vi "Module Init.vi"(8 "error in (no error)":errorcluster, 11 "ValveControlModule in":refnum<class "ValveControlModule.lvclass">) -> (0 "error out":errorcluster, 3 "ValveControlModule out":refnum<class "ValveControlModule.lvclass">)   [LabVIEW 2020, in "VolatusControl.lvlib" / "ValveControlModule.lvclass"]
uses:
  ValveControlModule.lvclass
  C:/dev/lv20CE/relink/lv-volatus/Volatus/Module/Module.lvclass
  Volatus/Remote Messaging Module/Message Registration.ctl
  lv-vecto/Vecto/Group/Group.lvclass
  C:/dev/lv20CE/relink/lv-vecto/Vecto/GroupAbstract/GroupAbstract.lvclass
  VolatusConfig/Meta Type.ctl
  Volatus/Module/Module.lvclass/Module.ctl
  VolatusConfig/VolatusConfigElement/VolatusConfigElement.lvclass/VolatusConfigElement.ctl
  ValveControlModule.lvclass/ValveControlModule.ctl
  Volatus/Module/Config.vi
  VolatusConfig/VolatusConfigElement/Element.vi
  VolatusConfig/Task/Task.lvclass
  C:/dev/lv20CE/relink/lv-volatus/VolatusConfig/VolatusConfigElement/VolatusConfigElement.lvclass
  lv-cdm/CDM-Config/Config Lookup/Match Meta.vi
  lv-cdm/CDM-Config/Config Element/Owner.vi
  lv-cdm/CDM-Config/Config Manager/Lookup Descendant.vi
  lv-cdm/CDM-Config/Config Filter/Config Lookup.lvclass
  lv-cdm/CDM-Config/Config Element/Config Element.lvclass
  Volatus/Module/Module.lvclass
  Volatus/Remote Messaging Module/Remote Messaging Module.lvclass
  VolatusConfig/Group/Group.lvclass
  VolatusData/Data Processor Module/Data Processor Module.lvclass
  C:/dev/lv20CE/relink/lv-volatus/VolatusControl/ValveControlModule/ValveControlModule.lvclass
  VolatusConfig/VolatusConfigElement/VolatusConfigElement.lvclass
  VolatusConfig/VolatusConfig.lvlib
  C:/dev/lv20CE/relink/lv-volatus/VolatusConfig/Task/Task.lvclass
  C:/dev/lv20CE/relink/lv-vecto/Vecto/Group/Group.lvclass
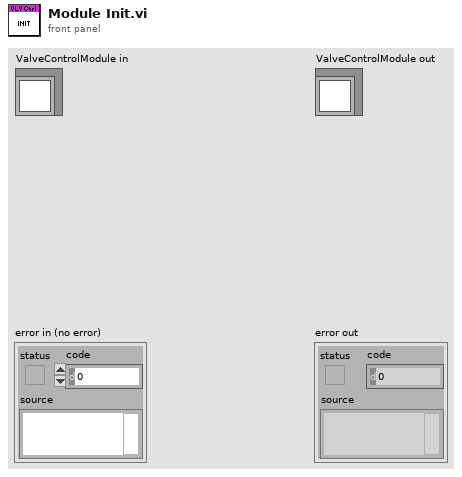
[diagram p1: front panel]
types:
  T1 = typedef "VolatusConfig.lvlib/Meta Type.ctl" = enum16{"UNKNOWN", "VL_System", "VL_Cluster", "VL_Node", "VL_Task", "VL_Group", "VL_Channel", "VL_Task_List", "VL_Scaling", "VL_Sensor", "VL_Sensor_List", "VL_Scale"}
  T2 = typedef "Volatus.lvlib/Remote Messaging Module.lvclass/Message Registration.ctl" = cluster{"Message Type":string, "Message ID":string}
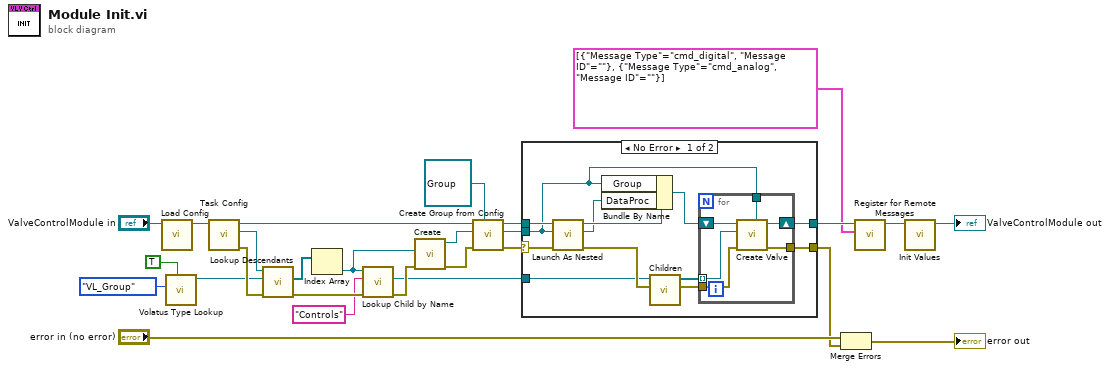
[diagram p0: block diagram]
diagram:
  n1 = call "Load Config.vi"("ValveControlModule in"="ValveControlModule in") -> ("ValveControlModule out"=w1:refnum<class "ValveControlModule.lvclass">)  [unwired: 9 in, 1 out]
  n2 = call "Volatus Type Lookup.vi"("Don't Recurse Past Match (F)"=TRUE, "Meta Type"=Meta_Type."VL_Group") -> ("Config Lookup out"=w8:refnum<class "Config Lookup.lvclass">)  [unwired: 8 in, 1 out]
  n3 = call "Task Config.vi"("Module in"=w1) -> ("error out"=w27:errorcluster, "Task Config"=w19:refnum<class "Task.lvclass">, "Module out"=w17:refnum<class "ValveControlModule.lvclass">)  [unwired: 8 in]
  n4 = call "Lookup Descendants.vi"("error in (no error)"=w27, "Lookup"=w8, "VolatusConfigElement in"=w19) -> ("error out"=w25:errorcluster, "Descendants"=w18:refnum<class "Config Element.lvclass">[])  [unwired: 6 in, 1 out]
  n5 = Index Array(array=w18) -> (element=w5:refnum<class "Config Element.lvclass">)  [unwired: 1 in]
  n6 = call "Lookup Child by Name.vi"("error in (no error)"=w25, "Name"="Controls", "Config Element in"=w5) -> ("error out"=w26:errorcluster, "Child"=w3:refnum<class "Config Element.lvclass">)  [unwired: 5 in, 2 out]
  n7 = call "Create.vi"("error in (no error)"=w26, "Element"=w5) -> ("error out"=w15:errorcluster, "Group out"=w16:refnum<class "Group.lvclass">)  [unwired: 8 in]
  n8 = call "Create Group from Config.vi"("Group Type (Abstract)"=refnum<class "Group.lvclass"> refnum ("Vecto.lvlib:Group.lvclass"), "error in (no error)"=w15, "Group Config"=w16, "Module in"=w17) -> ("error out"=w10:errorcluster, "Group"=w12:refnum<class "Group.lvclass">, "Module out"=w11:refnum<class "ValveControlModule.lvclass">)  [unwired: 5 in]
  n9 = case shown="No Error" w10 {
    selector: w10 -> [w30 w46]
    tunnel: [w36 w46] -> w21
    tunnel: w3 -> [w35 _]
    tunnel: [w34 w47] -> w13
    tunnel: w12 -> [w28 _]
    tunnel: w11 -> [w33 w47]
    frame No Error {
      n10 = call "Launch As Nested.vi"("error in (no error)"=w30, "Group"=w28, "Parent in"=w33) -> ("error out"=w39:errorcluster, "MessageQ"=w29:refnum<class "MessageQ.lvclass">, "Parent out"=w32:refnum<class "ValveControlModule.lvclass">)  [unwired: 6 in]
      n11 = Bundle By Name(cluster=w32, "Group"=w28, "DataProc"=w29) -> (w31:refnum<class "ValveControlModule.lvclass">)
      n12 = call "Children.vi"("error in (no error)"=w39, "Config Element in"=w35) -> ("error out"=w37:errorcluster, "Elements"=w38:refnum<class "Config Element.lvclass">[])  [unwired: 8 in]
      n13 = for {
        tunnel: w38 -> [w44] mode=indexing
        shift-right: [w43] -> w34
        shift-left: w31 -> [w45]
        tunnel: w37 -> [w42]
        tunnel: [w41] -> w36
        tunnel: w28 -> [w40]
        n14 = call "Create Valve.vi"("Group"=w40, "error in (no error)"=w42, "Config Element"=w44, "ValveControlModule in"=w45) -> ("error out"=w41:errorcluster, "ValveControlModule out"=w43:refnum<class "ValveControlModule.lvclass">)  [unwired: 6 in]
      }
    }
    frame Error {
    }
  }
  n15 = Merge Errors("error in (no error)", w21) -> (→"error out":errorcluster)
  n16 = call "Register for Remote Messages.vi"("Messages"=T2[] [{"Message Type"="cmd_digital", "Message ID"=""}, {"Message Type"="cmd_analog", "Message ID"=""}], "Module in"=w13) -> ("Module out"=w20:refnum<class "ValveControlModule.lvclass">)  [unwired: 8 in, 1 out]
  n17 = call "Init Values.vi"("ValveControlModule in"=w20) -> ("ValveControlModule out"=→"ValveControlModule out":refnum<class "ValveControlModule.lvclass">)  [unwired: 9 in, 1 out]
